vi "_PC_NS_SubVI_Signal_I162SGL.vi"(8 "error in (no error)":errorcluster, 10 "Int signal in":waveform(i16)) -> (0 "error out":errorcluster, 2 "dbl sigal out":waveform(dbl))   [LabVIEW 2016]
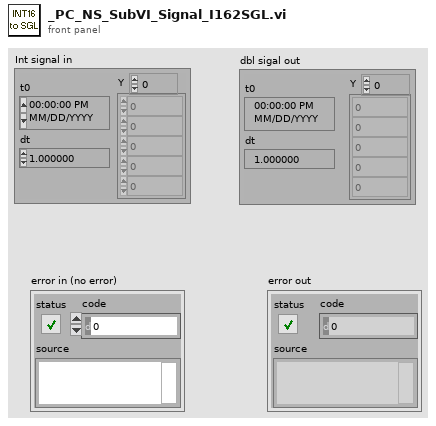
[diagram p1: front panel]
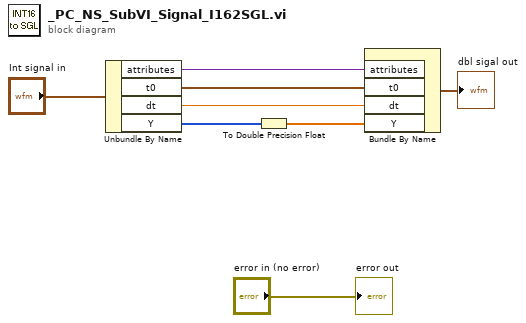
[diagram p0: block diagram]
diagram:
  n1 = Unbundle By Name("Int signal in") -> ("attributes"=w4:variant, "t0"=w5:timestamp, "dt"=w6:dbl, "Y"=w8:i16[])
  n2 = To Double Precision Float(number=w8) -> (double precision float=w2:dbl[])
  n3 = Bundle By Name("attributes"=w4, "t0"=w5, "dt"=w6, "Y"=w2) -> (→"dbl sigal out":waveform(dbl))  [unwired: 1 in]
  "error out" <- "error in (no error)"
